vi "Secure-Release Region.vi"(7 "Action":enum16{"Secure", "Release"}(ring), 8 "error in (no error)":errorcluster, 10 "Control In":T1={"I-O.lvclass"=refnum, "Gantry"=refnum, "Dispenser"="COM1"}, 11 "Carrier Tray in":refnum<class "Assembly Tray.lvclass">) -> (0 "error out":errorcluster, 1 "Position":i32, 2 "Control Out":T1={"I-O.lvclass"=refnum, "Gantry"=refnum, "Dispenser"="COM1"}, 3 "Carrier Tray out":refnum<class "Assembly Tray.lvclass">)   [LabVIEW 2021, in "Assembly Tray.lvclass"]
uses:
  Assembly Tray.lvclass
  C:/Users/HEP/Documents/GitHub/Gantry/UCSB-Gantry-HEP-main/Classes/Workspace/Fixture.lvclass
  Controller/Controllers.ctl
  Controller/I-O/I-O.lvclass
  C:/Program Files (x86)/Aerotech/A3200/LabVIEW/2010/Bin/Aerotech.A3200.dll
  Program Files (x86)/Aerotech/A3200/LabVIEW/2010/Bin/Aerotech.A3200.dll
  Fixture.lvclass/Fixture.ctl
  Assembly Tray.lvclass/Assembly Tray.ctl
  Fixture.lvclass
  Controller/Controller.lvclass
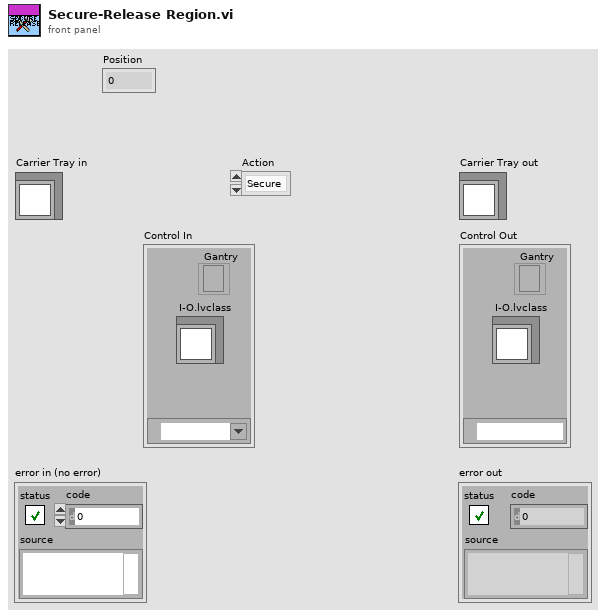
[diagram p1: front panel]
types:
  T1 = typedef "Controller.lvclass/Controllers.ctl" = cluster{"I-O.lvclass":refnum<class "I-O.lvclass">, "Gantry":refnum<k24>, "Dispenser":refnum<visa-resource-name>}
  T2 = typedef "I-O.lvclass/Pin Map.ctl" = cluster{"Region Valves":i32[], "Extra Valves":dbl[][][], "Tool Primary Valve":i32, "Tool Secondary Valve":i32, "Region Sensors":i32[], "Extra Sensors":dbl[][][], "Tool Primary Sensor":dbl, "Tool Secondary Sensor":dbl, "Compression Sensor":dbl, "5V":i32, "Dispenser Sensor":dbl}
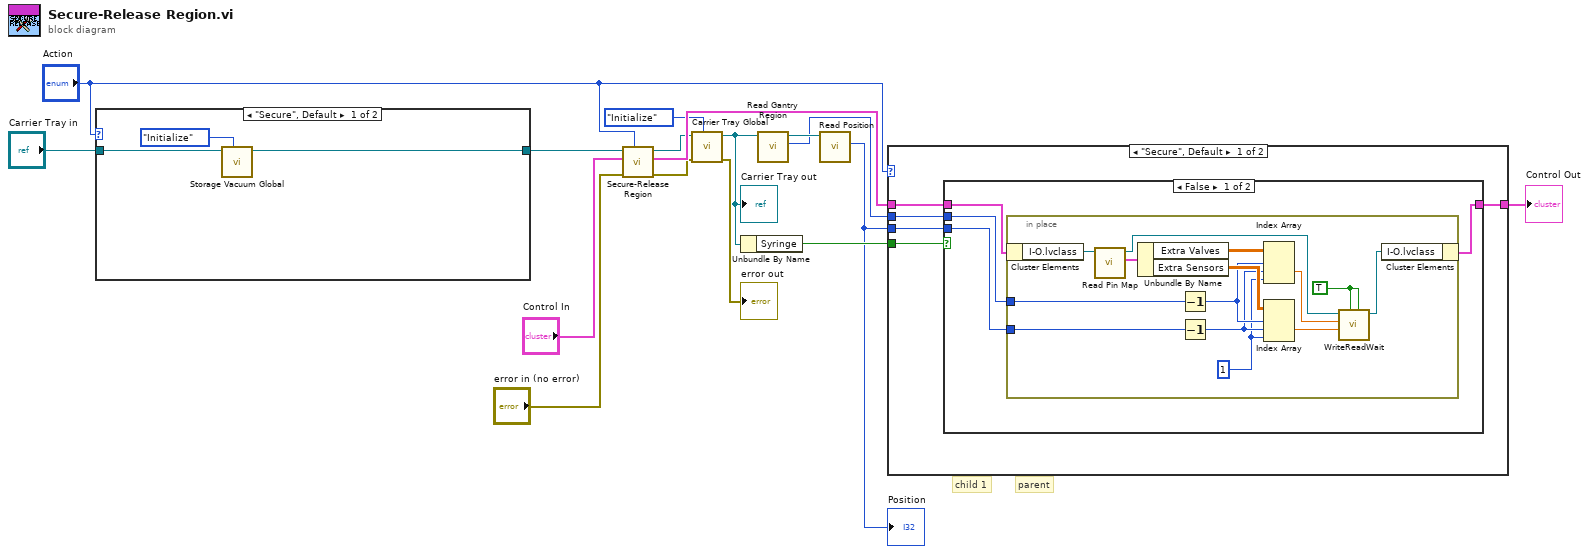
[diagram p0: block diagram]
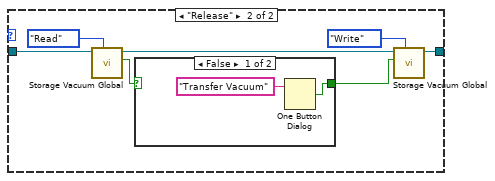
[diagram p4: hidden frame]
diagram:
  # "child 1"
  # "parent"
  n1 = case shown="\"Secure\", Default" "Action" {
    tunnel: [w18 w21] -> w13
    tunnel: "Carrier Tray in" -> [w17 w20]
    frame "Secure", Default {
      n2 = call "Storage Vacuum Global.vi"("Action"=enum16{"Initialize", "Read", "Write"}."Initialize", "Carrier Tray.lvclass"=w17) -> ("Carrier Tray.lvclass 2"=w18:refnum<class "Assembly Tray.lvclass">)  [unwired: 7 in, 2 out]
    }
    frame "Release" {
      n3 = call "Storage Vacuum Global.vi"("Action"=enum16{"Initialize", "Read", "Write"}."Read", "Carrier Tray.lvclass"=w20) -> ("Read"=w26:bool, "Carrier Tray.lvclass 2"=w22:refnum<class "Assembly Tray.lvclass">)  [unwired: 7 in, 1 out]
      n4 = case shown="False" w26 {
        selector: w26 -> [_ w29]
        tunnel: [w27 w29] -> w23
        frame False {
          n5 = One Button Dialog(message="Transfer Vacuum") -> (true=w27:bool)  [unwired: 1 in]
        }
        frame True {
        }
      }
      n6 = call "Storage Vacuum Global.vi"("Action"=enum16{"Initialize", "Read", "Write"}."Write", "Write"=w23, "Carrier Tray.lvclass"=w22) -> ("Carrier Tray.lvclass 2"=w21:refnum<class "Assembly Tray.lvclass">)  [unwired: 6 in, 2 out]
    }
  }
  n7 = call-parent "Secure-Release Region.vi"("Action"="Action", "error in (no error)"="error in (no error)", "Control In"="Control In", "Fixture in"=w13) -> ("error out"=w3:errorcluster, "Control Out"=w11:T1, "Fixture out"=w6:refnum<class "Assembly Tray.lvclass">)  [unwired: 4 in, 1 out]
  n8 = call "Carrier Tray Global.vi"("Action"=enum16{"Initialize", "Read", "Write"}."Initialize", "error in (no error)"=w3, "Carrier Tray.lvclass"=w6) -> ("error out"=→"error out":errorcluster, "Carrier Tray.lvclass 2"=w5:refnum<class "Assembly Tray.lvclass">)  [unwired: 6 in, 1 out]
  "Carrier Tray out" <- w5
  n9 = Unbundle By Name(w5) -> ("Syringe"=w12:bool)
  n10 = call "Read Gantry Region.vi"("Fixture in"=w5) -> ("Gantry Region"=w9:i32, "Fixture out"=w10:refnum<class "Assembly Tray.lvclass">)  [unwired: 8 in, 1 out]
  n11 = call "Read Position.vi"("Fixture in"=w10) -> ("Position"=w1:i32)  [unwired: 8 in, 2 out]
  "Position" <- w1
  n12 = case shown="\"Secure\", Default" "Action" {
    tunnel: w12 -> [w34 _]
    tunnel: w11 -> [w33 w54]
    tunnel: w9 -> [w32 _]
    tunnel: w1 -> [w31 _]
    tunnel: [w30 w54] -> w8
    frame "Secure", Default {
      n13 = case shown="False" w34 {
        tunnel: w33 -> [w38 w53]
        tunnel: w32 -> [w37 _]
        tunnel: w31 -> [w36 _]
        tunnel: [w35 w53] -> w30
        frame False {
          n14 = in-place {
            in-place-border: w37 -> [w46]
            in-place-border: w36 -> [w44]
            w42 = 1
            w48 = TRUE
            n15 = in-place-cluster #1(w38) -> ("I-O.lvclass"=w52:refnum<class "I-O.lvclass">)
            n16 = call-dynamic "Read Pin Map.vi"("I-O in"=w52) -> ("Pin Map 2"=w51:T2, "I-O out"=w49:refnum<class "I-O.lvclass">)  [unwired: 8 in, 1 out]
            n17 = Unbundle By Name(w51) -> ("Extra Valves"=w39:dbl[][][], "Extra Sensors"=w50:dbl[][][])
            n18 = Decrement(x=w46) -> (x-1=w45:i32)
            n19 = Decrement(x=w44) -> (x-1=w43:i32)
            n20 = Index Array(array=w39, index (dim 0)=w45, index (dim 1)=w43, index (dim 2)=w42) -> (element=w41:dbl)
            n21 = Index Array(array=w50, index (dim 0)=w45, index (dim 1)=w43, index (dim 2)=w42) -> (element=w40:dbl)
            n22 = call "WriteReadWait.vi"("Read Value"=w48, "Write Value"=w48, "Read"=w40, "Write"=w41, "I-O in"=w49) -> ("I-O out"=w47:refnum<class "I-O.lvclass">)  [unwired: 5 in, 1 out]
            n23 = in-place-cluster #1("I-O.lvclass"=w47) -> (w35:T1)
          }
        }
        frame True {
        }
      }
    }
    frame "Release" {
    }
  }
  "Control Out" <- w8
